vi "UnitTest-IsDataInserted.vi"(7 "Test Label":string="DB file has data Inserted in file separately", 8 "error in":errorcluster, 10 "Label (VI Title)":string="Backup on Launch - Unit Test I", 11 "TableLogger Config":T1={"TableLogger"=enum."CSV Logger", "DB File Path"=path "C:/LogAnyLVdata/Test.csv", "DB Backup Config"={"Directory"=path "C:/LogAnyLVdata/dBbackup", "UTC Time Format"=FALSE, "On Launch"=FALSE, "Interval (Hours)"=-1.0, "Size Multiples (Bytes)"=10000}}) -> (0 "error out":errorcluster)   [LabVIEW 2014]
uses:
  TableLogger_Actor/TableLoggerConfig.ctl
  TableLogger_Actor/TableLoggerTypes.ctl
  TableLogger_Actor/TableLoggerBackupConfig.ctl
  TableLogger_Actor/TableLoggerDataCluster.ctl
  TableLogger_Actor/Messages/InsertData_Msg/InsertData Msg.lvclass/InsertData Msg.ctl
  <vilib>/ActorFramework/Message Enqueuer/Message Enqueuer.lvclass/Message Enqueuer.ctl
  <vilib>/ActorFramework/Message Enqueuer/Enqueue.vi
  <vilib>/ActorFramework/Message Priority Queue/Priority Enqueue.vi
  TableLogger_Actor/Messages/InsertData_Msg/InsertData Msg.lvclass
  <vilib>/ActorFramework/Stop Msg/Stop Msg.lvclass
  <vilib>/addons/_JKI Toolkits/Caraya/classes/Assert/Assert.lvclass
  TableLogger_Actor/TableLogger_Actor/TableLogger_Actor.lvclass
  TableLogger_Actor/TableLogger_Actor.lvlib
  <vilib>/addons/_JKI Toolkits/Caraya/classes/Test/Test.lvclass
panel:
  # "Connector Pane"
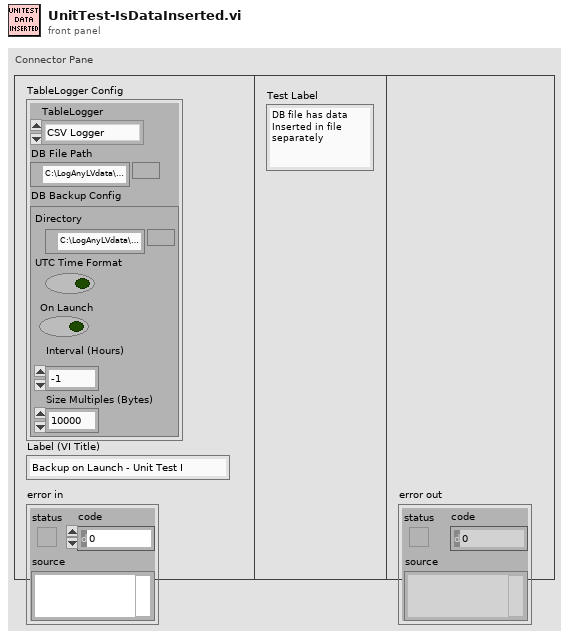
[diagram p1: front panel]
types:
  T1 = typedef "TableLogger_Actor.lvlib/TableLoggerConfig.ctl" = cluster{"TableLogger":T2, "DB File Path":path, "DB Backup Config":T3}
  T2 = typedef "TableLogger_Actor.lvlib/TableLoggerTypes.ctl" = enum16{"CSV Logger", "SQLite Logger"}
  T3 = typedef "TableLogger_Actor.lvlib/TableLoggerBackupConfig.ctl" = cluster{"Directory":path, "UTC Time Format":bool, "On Launch":bool, "Interval (Hours)":dbl, "Size Multiples (Bytes)":i32}
  T4 = typedef "TableLogger_Actor.lvlib/TableLoggerDataCluster.ctl" = cluster{"Numeric Data":i32, "Float Data":dbl, "String Data":string, "Enum Data":enum16{"Enum Item 1", "Enum Item 2"}, "Array Data":i32[]}
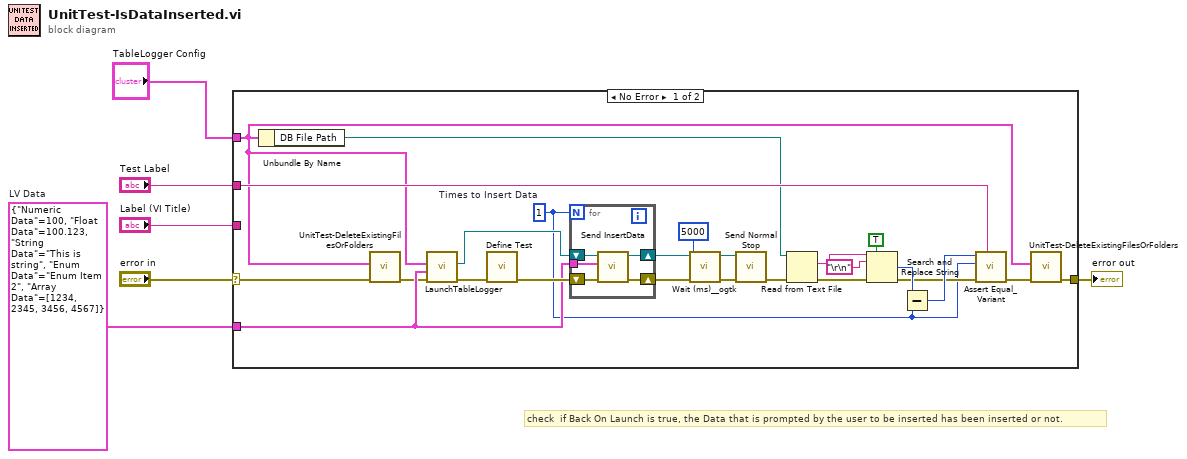
[diagram p0: block diagram]
diagram:
  w1 = T4 {"Numeric Data"=100, "Float Data"=100.123, "String Data"="This is string", "Enum Data"=enum."Enum Item 2", "Array Data"=[1234, 2345, 3456, 4567]}  # LV Data
  # "check  if Back On Launch is true, the Data that is prompted by the user to be inserted has been inserted or not."
  n1 = case shown="No Error" "error in" {
    selector: "error in" -> [w17 w36]
    tunnel: [w8 w36] -> w6
    tunnel: "TableLogger Config" -> [w9 _]
    tunnel: "Test Label" -> [w20 _]
    tunnel: "Label (VI Title)" -> [_ _]
    tunnel: w1 -> [w18 _]
    frame No Error {
      w7 = 1  # Times to Insert Data
      n2 = Unbundle By Name(w9) -> ("DB File Path"=w15:path)
      n3 = call "UnitTest-DeleteExistingFilesOrFolders.vi"("error in (no error)"=w17, "Config IN"=w9) -> ("error out"=w16:errorcluster)  [unwired: 9 in]
      n4 = call "LaunchTableLogger.vi"("error in (no error)"=w16, "Data Cluster (for Headers)"=w18, "TableLogger Config"=w9) -> ("error out"=w23:errorcluster, "TableLogger Actor's Enqueuer"=w19:refnum<class "Message Enqueuer.lvclass">)  [unwired: 5 in, 2 out]
      n5 = call <vilib>:"Define Test.vi"("error in (no error)"=w23) -> ("error out"=w22:errorcluster)  [unwired: 10 in]
      n6 = for {
        N: w7 -> [_]
        shift-right: [w34] -> w11
        shift-left: w22 -> [w35]
        shift-right: [w32] -> w13
        shift-left: w19 -> [w33]
        tunnel: w18 -> [w31]
        n7 = call "Send InsertData.vi"("error in (no error)"=w35, "Data"=w31, "Message Enqueuer"=w33) -> ("error out"=w34:errorcluster, "Message Enqueuer out"=w32:refnum<class "Message Enqueuer.lvclass">)  [unwired: 7 in]
      }
      n8 = call "Wait (ms)__ogtk.vi"("error in (no error)"=w11, "milliseconds to wait"=u32 5000) -> ("error out"=w10:errorcluster)  [unwired: 8 in, 1 out]
      n9 = call <vilib>:"Send Normal Stop.vi"("error in (no error)"=w10, "Message Enqueuer"=w13) -> ("error out"=w14:errorcluster)  [unwired: 9 in]
      n10 = Read from Text File(file (use dialog)=w15, error in=w14) -> (text=w24:string, error out=w30:errorcluster)  [unwired: 2 in, 2 out]
      n11 = Search and Replace String(replace all?=TRUE ("replace all? (F)"), input string=w24, search string="\r\n", error in=w30) -> (number of replacements=w27:i32, error out=w25:errorcluster)  [unwired: 4 in, 2 out]
      n12 = Subtract(x=w27, y=w7) -> (x-y=w26:i32)
      n13 = call <vilib>:"Assert Equal_Variant.vi"("Label"=w20, "error in (no error)"=w25, "Y"=w7, "X"=w26) -> ("error out"=w21:errorcluster)  [unwired: 7 in]
      n14 = call "UnitTest-DeleteExistingFilesOrFolders.vi"("error in (no error)"=w21, "Config IN"=w9) -> ("error out"=w8:errorcluster)  [unwired: 9 in]
    }
    frame Error {
    }
  }
  "error out" <- w6
